vi "Reinitialize.vi"(8 "error in (no error)":errorcluster, 11 "Arinst SSA-TG in":refnum<class "PL Arinst SSA-TG.lvclass">) -> (0 "error out":errorcluster, 3 "Arinst SSA-TG out":refnum<class "PL Arinst SSA-TG.lvclass">)   [LabVIEW 2015, in "PL Arinst SSA-TG.lvclass"]
doc: "Reinitializes connection to device based on previously specified settings."
uses:
  PL Arinst SSA-TG.lvclass
  PL Arinst SSA-TG.lvclass/PL Arinst SSA-TG.ctl
  <vilib>/Instr/_visa.llb/VISA Configure Serial Port (Instr).vi
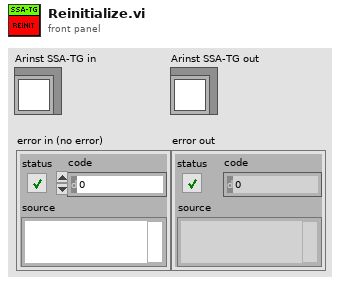
[diagram p1: front panel]
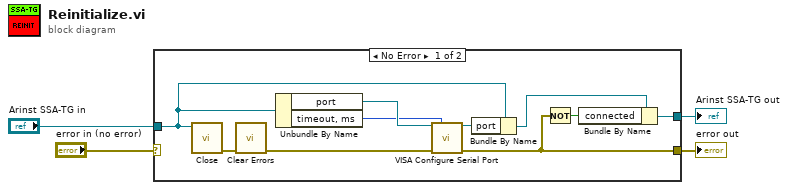
[diagram p0: block diagram]
diagram:
  n1 = case shown="No Error" "error in (no error)" {
    selector: "error in (no error)" -> [_ w15]
    tunnel: "Arinst SSA-TG in" -> [w14 w16]
    tunnel: [w11 w16] -> w3
    tunnel: [w6 w15] -> w2
    frame No Error {
      n2 = call "Close.vi"("Arinst SSA-TG in"=w14) -> ("error out"=w9:errorcluster)  [unwired: 10 in]
      n3 = call <vilib>:"Clear Errors.vi"("error in (no error)"=w9) -> ("error out"=w8:errorcluster)  [unwired: 5 in, 1 out]
      n4 = Unbundle By Name(w14) -> ("port"=w10:refnum<visa-resource-name>, "timeout, ms"=w5:u32)
      n5 = call-poly "VISA Configure Serial Port"("VISA resource name"=w10, "timeout (10sec)"=w5, "error in (no error)"=w8) -> ("VISA resource name out"=w7:refnum<visa-resource-name>, "error out"=w6:errorcluster)  [unwired: 11 in]
      n6 = Bundle By Name(cluster=w14, "port"=w7) -> (w13:refnum<class "PL Arinst SSA-TG.lvclass">)
      n7 = Not(x=w6) -> (.not. x?=w12:bool)
      n8 = Bundle By Name(cluster=w13, "connected"=w12) -> (w11:refnum<class "PL Arinst SSA-TG.lvclass">)
    }
    frame Error {
    }
  }
  "Arinst SSA-TG out" <- w3
  "error out" <- w2
